vi "Create Folder at Location.vi"(5 "Override existing":bool, 7 "Use Relative":bool, 8 "Error In":errorcluster, 10 "Path":string) -> (0 "Error Out":errorcluster, 2 "Full path out":path)   [LabVIEW 2019, in "VI Scripting Tools.lvlib"]
uses:
  VI Scripting Tools.lvlib
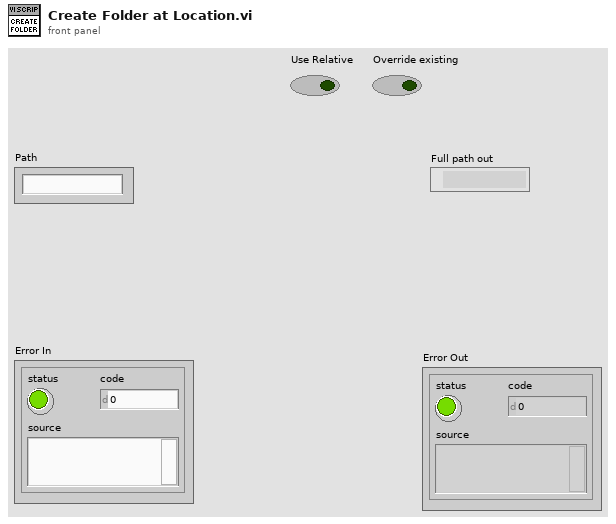
[diagram p1: front panel]
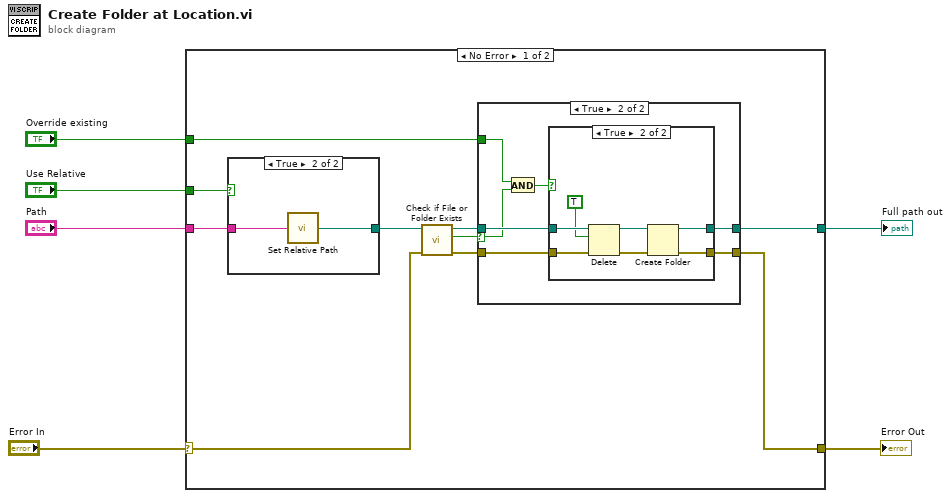
[diagram p0: block diagram]
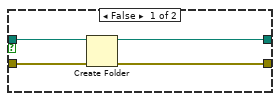
[diagram p2: hidden frame]
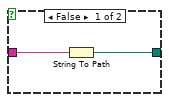
[diagram p4: hidden frame]
diagram:
  n1 = case shown="No Error" "Error In" {
    selector: "Error In" -> [w13 w41]
    tunnel: "Path" -> [w15 _]
    tunnel: "Use Relative" -> [w16 _]
    tunnel: "Override existing" -> [w9 _]
    tunnel: [w8 w41] -> w2
    tunnel: [w7 _] -> w1
    frame No Error {
      n2 = case shown="True" w16 {
        tunnel: w15 -> [w38 w40]
        tunnel: [w37 w39] -> w14
        frame False {
          n3 = String To Path(string=w38) -> (path=w37:path)
        }
        frame True {
          n4 = call "Set Relative Path.vi"("App Relative Path"=w40) -> ("Full Path"=w39:path)
        }
      }
      n5 = call <vilib>:"Check if File or Folder Exists.vi"("error in (no error)"=w13, "path"=w14) -> ("error out"=w10:errorcluster, "file or folder exists?"=w12:bool, "dup path"=w11:path)  [unwired: 7 in]
      n6 = case shown="True" w12 {
        selector: w12 -> [_ w25]
        tunnel: w11 -> [w19 w27]
        tunnel: w10 -> [w20 w23]
        tunnel: w9 -> [_ w26]
        tunnel: [w17 w22] -> w7
        tunnel: [w18 w21] -> w8
        frame False {
          n7 = Create Folder(path (use dialog)=w19, error in=w20) -> (created path=w17:path, error out=w18:errorcluster)  [unwired: 1 in, 1 out]
        }
        frame True {
          n8 = And(x=w26, y=w25) -> (x .and. y?=w24:bool)
          n9 = case shown="True" w24 {
            tunnel: w27 -> [w29 w36]
            tunnel: w23 -> [w28 w34]
            tunnel: [w28 w30] -> w21
            tunnel: [w29 w31] -> w22
            frame False {
            }
            frame True {
              n10 = Delete(path (use dialog)=w36, entire hierarchy (F)=TRUE, error in=w34) -> (deleted path=w32:path, error out=w33:errorcluster)  [unwired: 2 in, 1 out]
              n11 = Create Folder(path (use dialog)=w32, error in=w33) -> (created path=w31:path, error out=w30:errorcluster)  [unwired: 1 in, 1 out]
            }
          }
        }
      }
    }
    frame Error {
    }
  }
  "Error Out" <- w2
  "Full path out" <- w1
